vi "Get BuildSpec Version.vi"(8 "error in (no error)":errorcluster, 11 "Task in":refnum<class "Task.lvclass">) -> (0 "error out":errorcluster, 2 "BuildSpec Version":string, 3 "Task out":refnum<class "Task.lvclass">)   [LabVIEW 2017, in "Task Interface.lvlib" / "Task.lvclass"]
uses:
  Task.lvclass
  <vilib>/AppBuilder/AB_API_Simple/Build Specification Version.ctl
  <vilib>/AppBuilder/AB_API_Simple/NI_App_Builder_API.lvlib
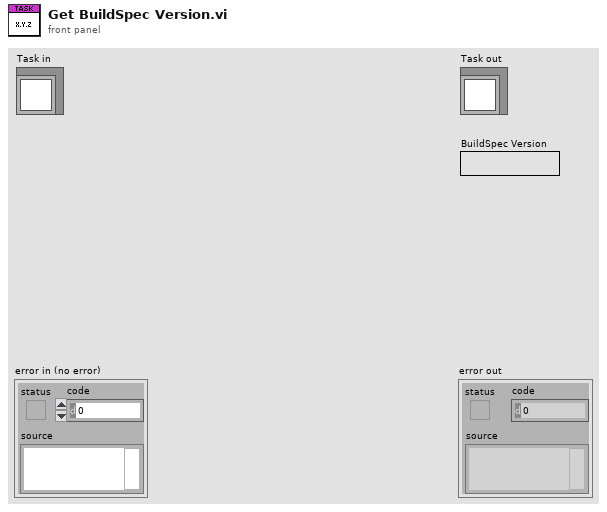
[diagram p1: front panel]
types:
  T1 = typedef "NI_App_Builder_API.lvlib/Build Specification Version.ctl" = cluster{"Major":u16, "Minor":u16, "Fix":u16, "Build":u16}
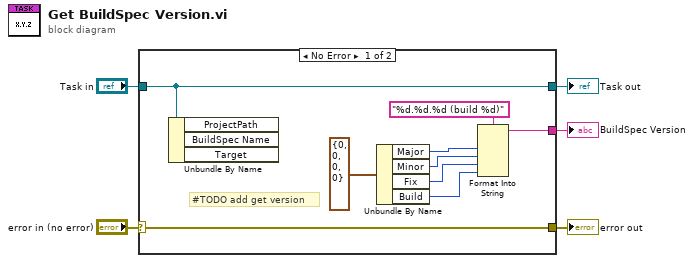
[diagram p0: block diagram]
diagram:
  n1 = case shown="No Error" "error in (no error)" {
    selector: "error in (no error)" -> [w13 w16]
    tunnel: [w13 w16] -> w4
    tunnel: [w14 w15] -> w2
    tunnel: "Task in" -> [w14 w15]
    tunnel: [w6 _] -> w1
    frame No Error {
      # "#TODO add get version"
      n2 = Unbundle By Name(w14) -> ()  [unwired: 3 out]
      n3 = Unbundle By Name(T1 {"Major"=0, "Minor"=0, "Fix"=0, "Build"=0} ("Build Specification Version")) -> ("Major"=w11:u16, "Minor"=w10:u16, "Fix"=w9:u16, "Build"=w8:u16)
      n4 = Format Into String(format string="%d.%d.%d (build %d)", w11, w10, w9, w8) -> (resulting string=w6:string)  [unwired: 2 in, 1 out]
    }
    frame Error {
    }
  }
  "error out" <- w4
  "Task out" <- w2
  "BuildSpec Version" <- w1
